vi "play_script.vi"(9 "Path Script":path, 11 "Connection":cluster{"queue out":refnum<queue>}) -> (3 "Connection":cluster{"queue out":refnum<queue>})   [LabVIEW 2019]
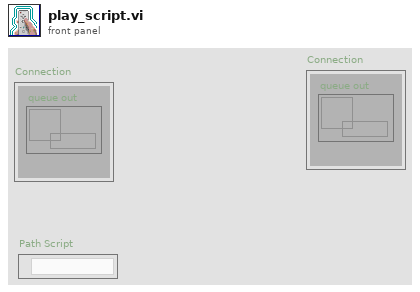
[diagram p1: front panel]
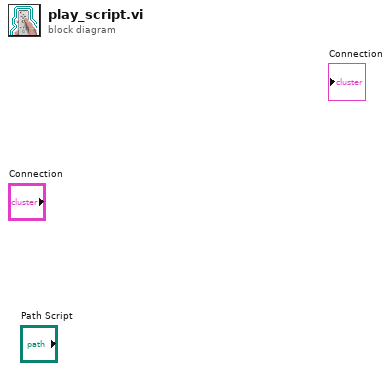
[diagram p0: block diagram]
diagram:
